vi "AP2x4x SetCenterWavelenghtOrFrequency.vi"(6 "Unit":enum16{"Wavelenght", "Frequency"}(ring), 7 "Center":dbl, 8 "error in":errorcluster, 11 "AP2x4x IN":refnum<visa-resource-name>="TCPIP0::169.254.53.138::5900::SOCKET") -> (0 "error out":errorcluster, 3 "AP2x4x OUT":refnum<visa-resource-name>="TCPIP0::169.254.53.138::5900::SOCKET")   [LabVIEW 2014]
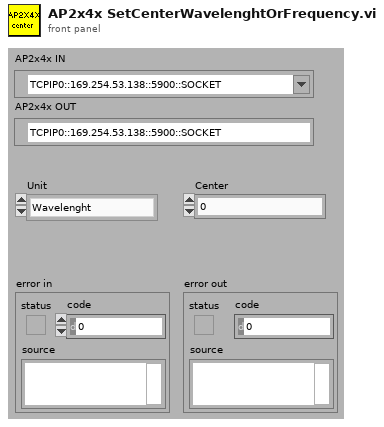
[diagram p1: front panel]
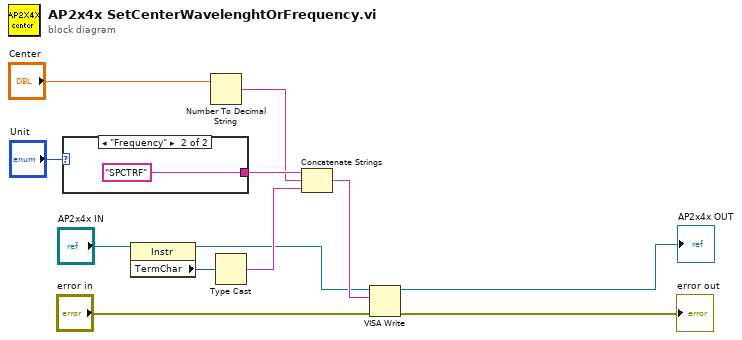
[diagram p0: block diagram]
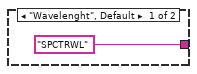
[diagram p2: hidden frame]
diagram:
  n1 = case shown="\"Frequency\"" "Unit" {
    tunnel: ["SPCTRWL" ("data string") "SPCTRF" ("data string")] -> w11
    frame "Wavelenght", Default {
    }
    frame "Frequency" {
    }
  }
  n2 = property class="Instr"(reference="AP2x4x IN") -> (reference out=w6:refnum<visa-resource-name>, "TermChar"=w9:u8)  [unwired: 1 in, 1 out]
  n3 = Number To Decimal String(number="Center") -> (decimal integer string=w5:string)  [unwired: 1 in]
  n4 = Type Cast(x=w9) -> (*(type *) &x=w8:string)  [unwired: 1 in]
  n5 = Concatenate Strings(w11, w5, w8) -> (w10:string)
  n6 = VISA Write(VISA resource name=w6, write buffer=w10, error in (no error)="error in") -> (VISA resource name out=→"AP2x4x OUT":refnum<visa-resource-name>, error out=→"error out":errorcluster)  [unwired: 1 out]
